vi "resources.vi"() -> ()   [LabVIEW 2013]
panel:
  out "CY semaphore":T1
  out "CX semaphore":T1
  out "DI semaphore":T1
  out "AI semaphore":T1
  out "monitor event":refnum<user-event>
  out "notifier":refnum<notifier>
  out "cmd queue":refnum<queue>
  out "tasks":T2
  out "motor status event":refnum<user-event>
  out "motor move event":refnum<user-event>
  out "user event":refnum<user-event>
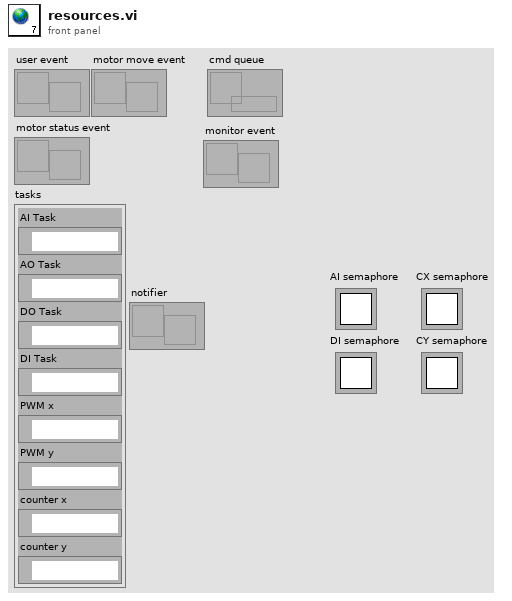
[diagram p1: front panel]
types:
  T1 = typedef "Semaphore RefNum" = refnum<k1>
  T2 = cluster{"AI Task":refnum<k21>, "AO Task":refnum<k21>, "DO Task":refnum<k21>, "DI Task":refnum<k21>, "PWM x":refnum<k21>, "PWM y":refnum<k21>, "counter x":refnum<k21>, "counter y":refnum<k21>}
diagram:
